vi "Scan Engine-Single Frame.vi"(7 "Channel":u32(ring)=1 items=["A"=1, "B"=2, "A + B"=3, "C"=4, "A + C"=5, "A + B"=6, "D"=8, "A + D"=9, "B + D"=10, "C + D"=12, "A + B + C + D"=15], 8 "Error in":errorcluster, 10 "Scan Status":enum16{"Start", "Continue Scan", "Finish Scan"}(ring)=enum."Continue Scan") -> (0 "Error Out":errorcluster, 1 "Return Code":u32, 3 "data out float":sgl[](array[numeric]), 4 "Data out U16":u16[](array[numeric]))   [LabVIEW 2018]
uses:
  Hardware Mfg/AlazarTech SDK/Controls/Alazar Engine Actions.ctl
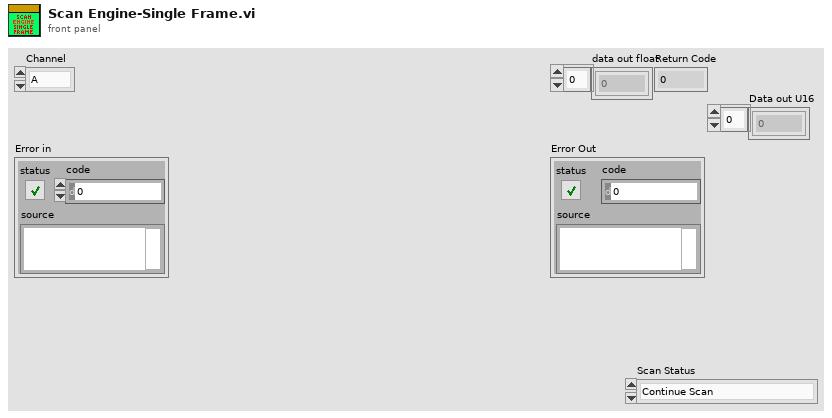
[diagram p1: front panel]
types:
  T1 = typedef "Alazar Engine Actions.ctl" = enum16{"Init", "Config Clock", "Config Ch", "Config Trig", "Config Non-FFT Acq.", "Non-FFT Acquire", "Load background from Non-FFT buffer", "enable background subtrac", "disable background subtrac", "load background from file", "load background from elsewhere", "start acquire", "background subtraction", "Config Acq.", "Acquire", "UnInit"}
  T2 = enum16{"Configure channels", "Write Scan Pattern", "Start Galvo Task", "Is Task Done?", "Stop Galvo", "Uninit", "Init: Calc scan pattern"}
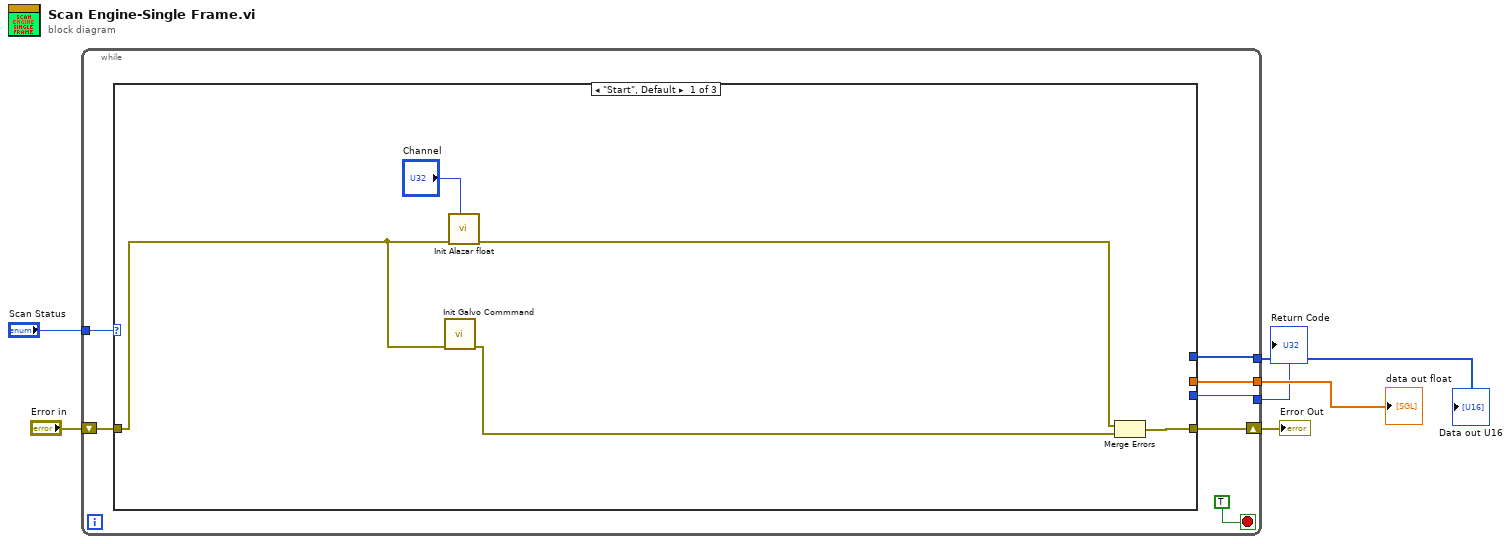
[diagram p0: block diagram]
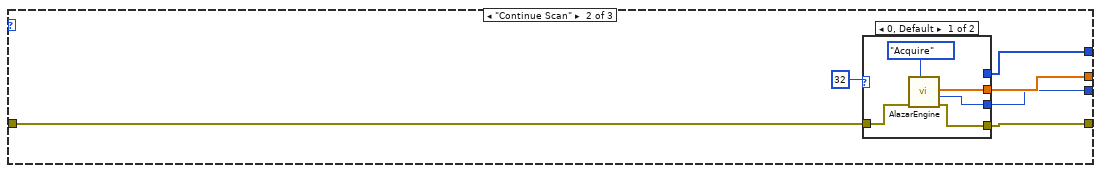
[diagram p2: hidden frame]
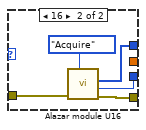
[diagram p3: hidden frame]
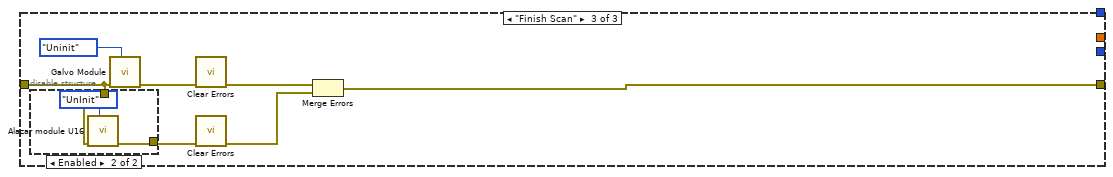
[diagram p4: hidden frame]
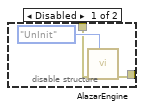
[diagram p5: hidden frame]
diagram:
  n1 = while {
    shift-right: [w12] -> w5
    shift-left: "Error in" -> [w10]
    tunnel: "Scan Status" -> [w11]
    tunnel: [w9] -> w3
    tunnel: [w8] -> w2
    tunnel: [w7] -> w1
    stop <- TRUE ("Status In") stop-if-true
    n2 = case shown="\"Start\", Default" w11 {
      tunnel: w10 -> [w17 w22 w38]
      tunnel: [w18 w19 w35] -> w12
      tunnel: [_ w24 _] -> w9
      tunnel: [_ w23 _] -> w8
      tunnel: [_ w20 _] -> w7
      frame "Start", Default {
        n3 = call "Init Galvo Commmand.vi"("error in (no error)"=w17) -> ("error out"=w15:errorcluster)  [unwired: 10 in]
        n4 = call "Init Alazar float.vi"("Channel"="Channel", "error in (no error)"=w17) -> ("error out"=w16:errorcluster)  [unwired: 9 in]
        n5 = Merge Errors(w16, w15) -> (w18:errorcluster)
      }
      frame "Continue Scan" {
        n6 = case shown="0, Default" 32 {
          tunnel: [w26 _] -> w24
          tunnel: [w27 w34] -> w23
          tunnel: w22 -> [w29 w33]
          tunnel: [w28 w32] -> w19
          tunnel: [_ w30] -> w20
          frame 0, Default {
            n7 = call "AlazarEngine.vi"("Action"=Alazar_Engine_Actions."Acquire", "error in (no error)"=w29) -> ("error out"=w28:errorcluster, "Return Code"=w27:u32, "Buffer"=w26:sgl[])  [unwired: 7 in]
          }
          frame 16 {
            n8 = call "Alazar module U16.vi"("Action"=Alazar_Engine_Actions."Acquire", "error in (no error)"=w33) -> ("error out"=w32:errorcluster, "Return Code"=w34:u32, "Buffer"=w30:u16[])  [unwired: 7 in]
          }
        }
      }
      frame "Finish Scan" {
        n9 = disable-structure shown="Enabled" {
          disable-tunnel: [w43 w46] -> w40
          disable-tunnel: w38 -> [w42 w47]
          frame Disabled {
            n10 = call "AlazarEngine.vi"("Action"=Alazar_Engine_Actions."UnInit", "error in (no error)"=w42) -> ("error out"=w43:errorcluster)  [unwired: 7 in, 2 out]
          }
          frame Enabled {
            n11 = call "Alazar module U16.vi"("Action"=Alazar_Engine_Actions."UnInit", "error in (no error)"=w47) -> ("error out"=w46:errorcluster)  [unwired: 7 in, 2 out]
          }
        }
        n12 = call "Galvo Module.vi"("Action"=T2."Uninit", "error in (no error)"=w38) -> ("error out"=w41:errorcluster)  [unwired: 8 in, 1 out]
        n13 = call <vilib>:"Clear Errors.vi"("error in (no error)"=w41) -> ("error out"=w37:errorcluster)  [unwired: 5 in, 1 out]
        n14 = call <vilib>:"Clear Errors.vi"("error in (no error)"=w40) -> ("error out"=w36:errorcluster)  [unwired: 5 in, 1 out]
        n15 = Merge Errors(w37, w36) -> (w35:errorcluster)
      }
    }
  }
  "Error Out" <- w5
  "data out float" <- w3
  "Return Code" <- w2
  "Data out U16" <- w1
